vi "Global Variable.vi"() -> ()   [LabVIEW 2018]
panel:
  out "SIM-SIS-RX-ARRAY":bool[](array[boolean])
  out "SIM-BPCS-RX-ARRAY":dbl[](array[numeric])
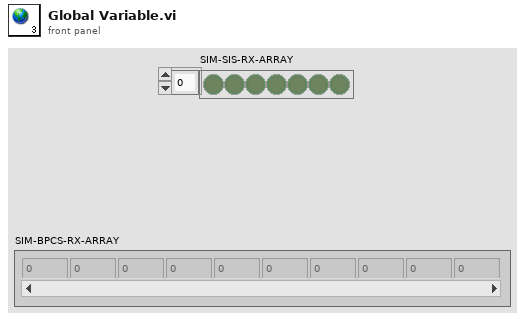
[diagram p1: front panel]
diagram:
